vi "SaveStatsIntoDB.vi"(8 "error in (no error)":errorcluster, 11 "ClashRoyale in":refnum<class "StashRoyale.lvclass">) -> (0 "error out":errorcluster, 3 "ClashRoyale out":refnum<class "StashRoyale.lvclass">)   [LabVIEW 2020, in "StashRoyale.lvclass"]
uses:
  StashRoyale.lvclass
  StashRoyale.lvclass/StashRoyale.ctl
  <vilib>/drjdpowell/SQLite Library/SQL Connection/Execute SQL (No results).vi
  <vilib>/drjdpowell/SQLite Library/SQLite.lvlib
  <vilib>/drjdpowell/SQLite Library/SQL Connection/Connection.lvclass
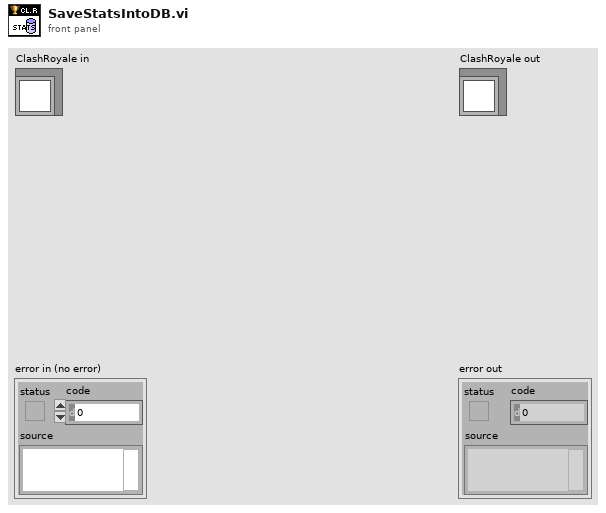
[diagram p1: front panel]
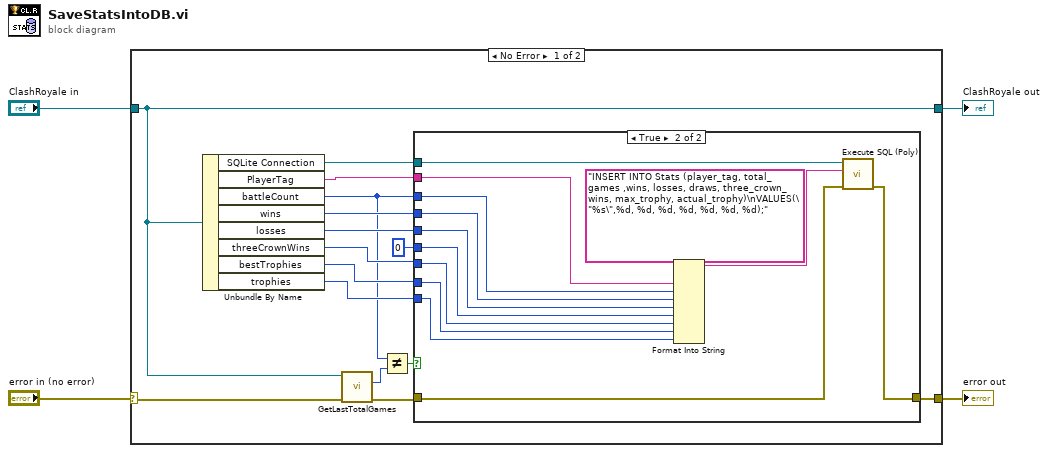
[diagram p0: block diagram]
diagram:
  n1 = case shown="No Error" "error in (no error)" {
    selector: "error in (no error)" -> [w10 w35]
    tunnel: [w14 w35] -> w3
    tunnel: [w11 w34] -> w1
    tunnel: "ClashRoyale in" -> [w11 w34]
    frame No Error {
      n2 = Unbundle By Name(w11) -> ("SQLite Connection"=w19:refnum<class "Connection.lvclass">, "PlayerTag"=w18:string, "battleCount"=w7:u16, "wins"=w17:u16, "losses"=w16:u16, "threeCrownWins"=w15:u16, "bestTrophies"=w13:u16, "trophies"=w12:u16)
      n3 = call "GetLastTotalGames.vi"("error in (no error)"=w10, "ClashRoyale in"=w11) -> ("error out"=w9:errorcluster, "Last Total Games"=w8:i64)  [unwired: 7 in, 1 out]
      n4 = Not Equal?(x=w7, y=w8) -> (x != y?=w6:bool)
      n5 = case shown="True" w6 {
        tunnel: w19 -> [_ w33]
        tunnel: w18 -> [_ w31]
        tunnel: w7 -> [_ w30]
        tunnel: w17 -> [_ w29]
        tunnel: w16 -> [_ w28]
        tunnel: u32 0 ("1v1 draws") -> [_ w27]
        tunnel: w15 -> [_ w26]
        tunnel: w9 -> [w20 w24]
        tunnel: [w20 w23] -> w14
        tunnel: w13 -> [_ w22]
        tunnel: w12 -> [_ w21]
        frame False {
          # "Pas de nouvelles parties jouées"
        }
        frame True {
          n6 = Format Into String(format string="INSERT INTO Stats (player_tag, total_games ,wins, losses, draws, three_crown_wins, max_trophy, actual_trophy)\nVALUES(\"%s\",%d, %d, %d, %d, %d, %d, %d);", w31, w30, w29, w28, w27, w26, w22, w21) -> (resulting string=w25:string)  [unwired: 2 in, 1 out]
          n7 = call-poly <vilib>:"Execute SQL (Poly).vi"("error in (no error)"=w24, "SQL"=w25, "SQLite Connection in"=w33) -> ("error out"=w23:errorcluster)  [unwired: 7 in, 1 out]
        }
      }
    }
    frame Error {
    }
  }
  "error out" <- w3
  "ClashRoyale out" <- w1
